vi "Read_Left_Joint_Notifier.vi"(5 "error in":errorcluster, 8 "ignore previous (F)":bool) -> (0 "error out":errorcluster, 3 "Positions":dbl[](array[numeric]) format="%.3f")   [LabVIEW 2013]
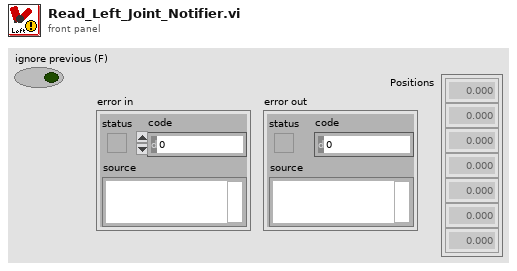
[diagram p1: front panel]
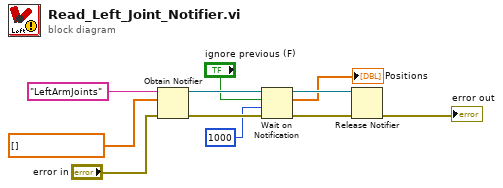
[diagram p0: block diagram]
diagram:
  n1 = Obtain Notifier(name (unnamed)="LeftArmJoints", notification data type=dbl[] [], error in (no error)="error in") -> (notifier out=w10:refnum<notifier>, error out=w5:errorcluster)  [unwired: 1 in, 1 out]
  n2 = Wait on Notification(notifier=w10, ignore previous (F)="ignore previous (F)", timeout in ms (-1)=1000, error in (no error)=w5) -> (notifier out=w8:refnum<notifier>, notification=→"Positions":dbl[], error out=w6:errorcluster)  [unwired: 1 out]
  n3 = Release Notifier(notifier=w8, error in (no error)=w6) -> (error out=→"error out":errorcluster)  [unwired: 1 in, 2 out]
